vi "Compute Time Remaining.vi"(8 "error in (no error)":errorcluster, 11 "Dialog in":refnum<class "Dialog.lvclass">) -> (0 "error out":errorcluster, 1 "Elapsed":bool, 2 "Time remaining (s)":dbl, 3 "Dialog out":refnum<class "Dialog.lvclass">)   [LabVIEW 2012, in "Dialog.lvlib" / "Dialog.lvclass"]
uses:
  Dialog.lvclass
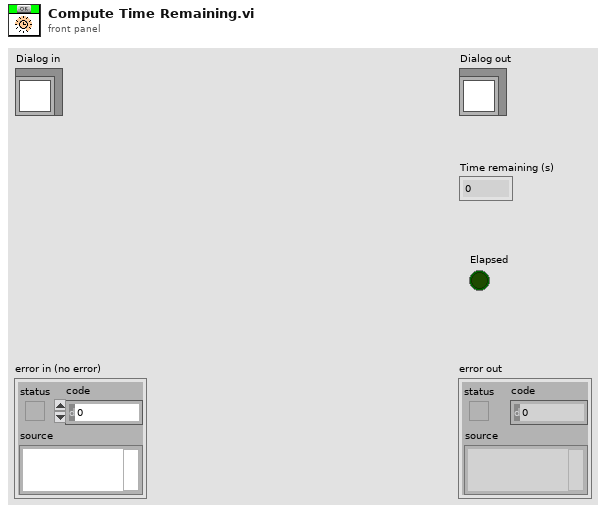
[diagram p1: front panel]
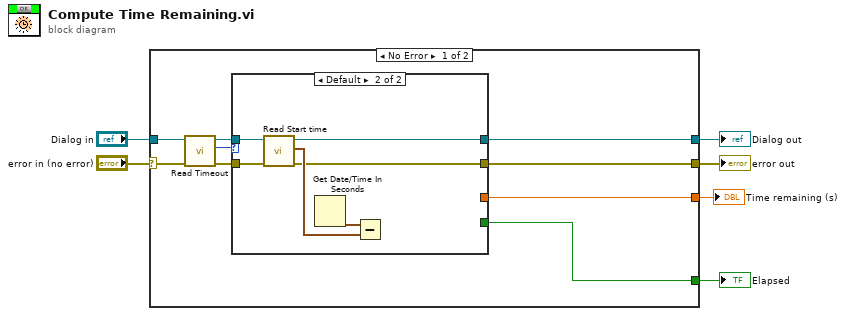
[diagram p0: block diagram]
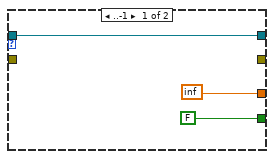
[diagram p2: hidden frame]
diagram:
  n1 = case shown="No Error" "error in (no error)" {
    selector: "error in (no error)" -> [w8 w26]
    tunnel: [w7 w26] -> w5
    tunnel: [w13 w25] -> w3
    tunnel: "Dialog in" -> [w15 w25]
    tunnel: [w11 _] -> w2
    tunnel: [w10 _] -> w1
    frame No Error {
      n2 = call-dynamic "Read Timeout.vi"("error in (no error)"=w8, "Dialog.lvclass in"=w15) -> ("error out"=w9:errorcluster, "Timeout"=w12:i32, "Dialog.lvclass out"=w14:refnum<class "Dialog.lvclass">)  [unwired: 7 in]
      n3 = case shown="Default" w12 {
        tunnel: w14 -> [w18 w24]
        tunnel: [w18 w23] -> w13
        tunnel: [FALSE _] -> w11
        tunnel: [inf _] -> w10
        tunnel: w9 -> [_ w20]
        tunnel: [_ w19] -> w7
        frame ..-1 {
        }
        frame Default {
          n4 = call "Read Start time.vi"("error in (no error)"=w20, "Dialog in"=w24) -> ("error out"=w19:errorcluster, "Start time"=w22:timestamp, "Dialog out"=w23:refnum<class "Dialog.lvclass">)  [unwired: 7 in]
          n5 = Get Date/Time In Seconds() -> (seconds since 1Jan1904=w21:timestamp)
          n6 = Subtract(x=w21, y=w22) -> ()  [unwired: 1 out]
        }
      }
    }
    frame Error {
    }
  }
  "error out" <- w5
  "Dialog out" <- w3
  "Time remaining (s)" <- w1
  "Elapsed" <- w2
